vi "ConvertTimes - Single.vi"(1 "GP22 Output":u32) -> (0 "Time/s":dbl)   [LabVIEW 2013, in "GP22_TDC_Arduinoed.lvlib"]
doc: "Convert fixed point output of GP22 to time value in seconds. \n\nDepending on whether the TDC is in calibration mode or not, adjust the raw data by either the Ref clock's period (calibrated mode) or the calibration LSB time (uncalibrated mode)."
uses:
  GP22_TDC_Arduinoed.lvlib
  Public/Globals.vi
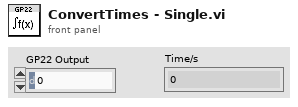
[diagram p1: front panel]
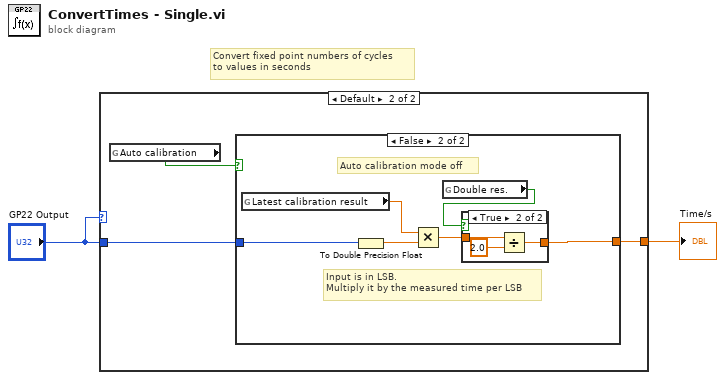
[diagram p0: block diagram]
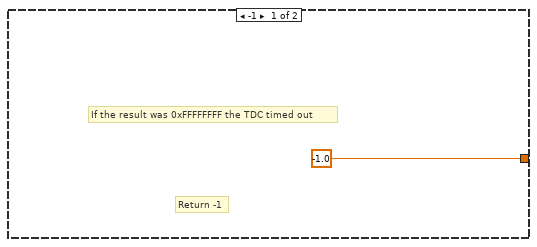
[diagram p2: hidden frame]
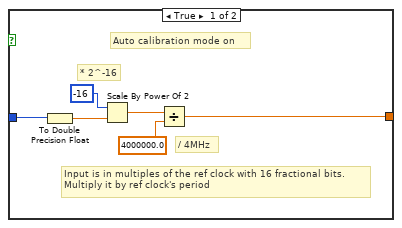
[diagram p3: hidden frame]
diagram:
  # "Convert fixed point numbers of cycles\nto values in seconds"
  n1 = case shown="Default" "GP22 Output" {
    tunnel: [-1.0 w6] -> w2
    tunnel: "GP22 Output" -> [_ w5]
    frame -1 {
      # "Return -1"
      # "If the result was 0xFFFFFFFF the TDC timed out"
    }
    frame Default {
      n2 = global read "Globals.vi" "Auto calibration"() -> (w4:bool)
      n3 = case shown="False" w4 {
        tunnel: [w10 w15] -> w6
        tunnel: w5 -> [w8 w18]
        frame True {
          # "Input is in multiples of the ref clock with 16 fractional bits.\nMultiply it by ref clock's period"
          # "Auto calibration mode on"
          # "/ 4MHz"
          # "* 2^-16"
          n4 = To Double Precision Float(number=w8) -> (double precision float=w7:dbl)
          n5 = Scale By Power Of 2(n=i16 -16, x=w7) -> (x*2^n=w11:dbl)
          n6 = Divide(x=w11, y=4000000.0) -> (x/y=w10:dbl)
        }
        frame False {
          # "Input is in LSB. \nMultiply it by the measured time per LSB"
          # "Auto calibration mode off"
          n7 = global read "Globals.vi" "Latest calibration result"() -> (w16:dbl)
          n8 = To Double Precision Float(number=w18) -> (double precision float=w17:dbl)
          n9 = Multiply(x=w16, y=w17) -> (x*y=w14:dbl)
          n10 = global read "Globals.vi" "Double res."() -> (w13:bool)
          n11 = case shown="True" w13 {
            tunnel: [w19 w22] -> w15
            tunnel: w14 -> [w19 w21]
            frame False {
            }
            frame True {
              n12 = Divide(x=w21, y=2.0) -> (x/y=w22:dbl)
            }
          }
        }
      }
    }
  }
  "Time/s" <- w2
